vi "Link Bone Communication.vi"(6 "VISA resource name":refnum<visa-resource-name>="COM3", 8 "error in":errorcluster, 11 "Commands":string[](array[string])=["reset", "on A, I", "on B, J", "on C, K"]) -> (0 "error out":errorcluster)   [LabVIEW 2012]
uses:
  <vilib>/Instr/_visa.llb/VISA Configure Serial Port (Instr).vi
panel:
  out "read buffer":string
  out "Numeric":i32
  out "concatenated string":string
  out "bytes read":u32
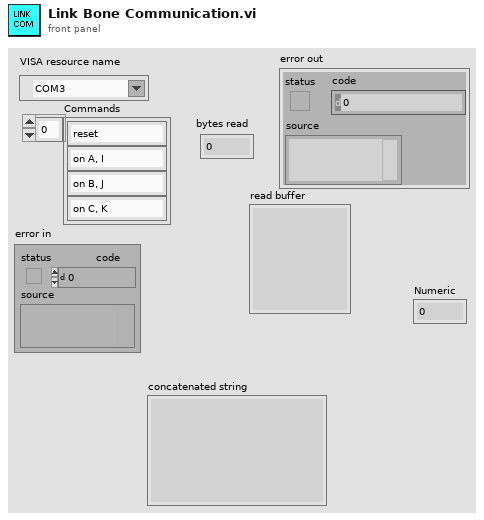
[diagram p1: front panel]
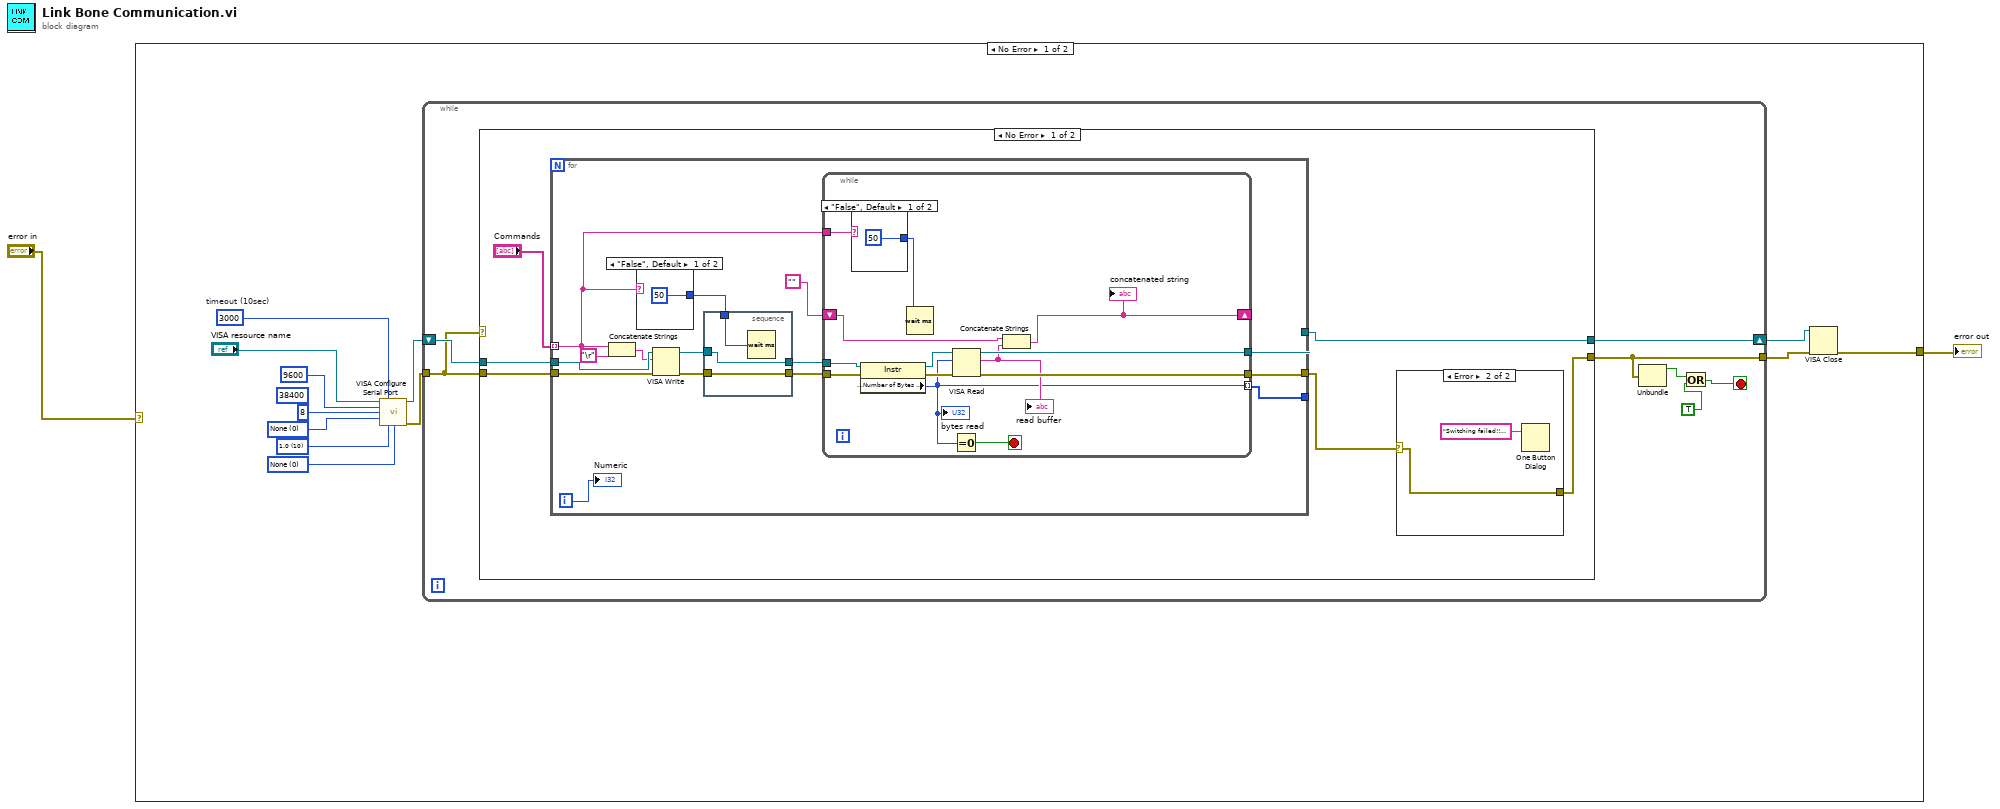
[diagram p0: block diagram]
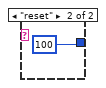
[diagram p3: hidden frame]
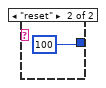
[diagram p4: hidden frame]
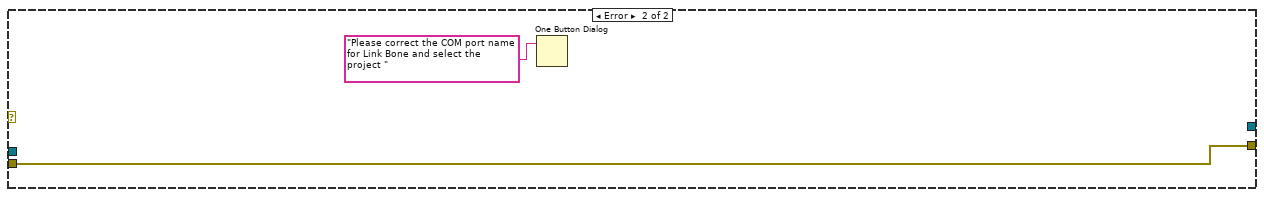
[diagram p5: hidden frame]
diagram:
  n1 = case shown="No Error" "error in" {
    selector: "error in" -> [_ w68]
    tunnel: [w3 w68] -> w1
    frame No Error {
      w6 = u16 0 items=["None"=0, "XON/XOFF"=1, "RTS/CTS"=2, "DTR/DSR"=4] ("flow control")
      w7 = u16 10 items=["1.0"=10, "1.5"=15, "2.0"=20] ("stop bits")
      w9 = u16 0 items=["None", "Odd", "Even", "Mark", "Space"] ("parity")
      (unwired) u32 38400 ("baud rate")
      w8 = u32 3000  # timeout (10sec)
      n2 = call-poly "VISA Configure Serial Port"("VISA resource name"="VISA resource name", "timeout (10sec)"=w8, "baud rate (9600)"=u32 9600 ("baud rate"), "data bits (8)"=u16 8 ("data bits"), "parity (0:none)"=w9, "stop bits (10: 1 bit)"=w7, "flow control (0:none)"=w6) -> ("VISA resource name out"=w12:refnum<visa-resource-name>, "error out"=w13:errorcluster)  [unwired: 2 in, 5 out]
      n3 = while {
        tunnel: w13 -> [w16]
        tunnel: [w15] -> w11
        shift-right: [w20] -> w10
        shift-left: w12 -> [w21]
        stop <- w18 stop-if-true
        n4 = case shown="No Error" w16 {
          tunnel: w16 -> [w27 w66]
          tunnel: w21 -> [w26 _]
          tunnel: [w25 _] -> w20
          tunnel: [w23 w66] -> w15
          frame No Error {
            n5 = for {
              tunnel: w27 -> [w45]
              tunnel: w26 -> [w44]
              tunnel: [w31] -> w22
              tunnel: [w43] -> w25
              tunnel: "Commands" -> [w33] mode=indexing
              tunnel: [w32] -> _
              i -> [w35]
              n6 = Concatenate Strings(w33, "\r") -> (w37:string)
              n7 = case shown="\"False\", Default" w33 {
                tunnel: [u32 50 ("delay before read (ms)") u32 100 ("delay before read (ms)")] -> w34
                frame "False", Default {
                }
                frame "reset" {
                }
              }
              n8 = VISA Write(VISA resource name=w44, write buffer=w37, error in (no error)=w45) -> (VISA resource name out=w40:refnum<visa-resource-name>, error out=w42:errorcluster)  [unwired: 1 out]
              n9 = stacked-sequence {
                tunnel: w42 -> [w65]
                tunnel: [w65] -> w41
                tunnel: w40 -> [w64]
                tunnel: [w64] -> w39
                tunnel: w34 -> [w63]
                frame #0 {
                  n10 = Wait (ms)(milliseconds to wait=w63) -> ()  [unwired: 1 out]
                }
              }
              n11 = while {
                tunnel: [w60] -> w31
                tunnel: [w59] -> w43
                tunnel: w41 -> [w58]
                tunnel: w39 -> [w57]
                shift-right: [w51] -> _
                shift-left: "" -> [w53]
                tunnel: w33 -> [w49]
                tunnel: [w48] -> w32 mode=indexing
                stop <- w54 stop-if-true
                n12 = case shown="\"False\", Default" w49 {
                  tunnel: [u32 50 ("delay before read (ms)") u32 100 ("delay before read (ms)")] -> w50
                  frame "False", Default {
                  }
                  frame "reset" {
                  }
                }
                n13 = property class="Instr"(reference=w57, error in=w58) -> (reference out=w56:refnum<visa-resource-name>, error out=w55:errorcluster, "Serial Settings:Number of Bytes at Serial Port"=w48:u32)
                "bytes read" <- w48
                n14 = Wait (ms)(milliseconds to wait=w50) -> ()  [unwired: 1 out]
                n15 = VISA Read(VISA resource name=w56, byte count=w48, error in (no error)=w55) -> (VISA resource name out=w59:refnum<visa-resource-name>, read buffer=w52:string, error out=w60:errorcluster)  [unwired: 1 out]
                "read buffer" <- w52
                n16 = Equal To 0?(x=w48) -> (x = 0?=w54:bool)
                n17 = Concatenate Strings(w53, w52) -> (w51:string)
                "concatenated string" <- w51
              }
              "Numeric" <- w35
            }
            n18 = case shown="Error" w22 {
              selector: w22 -> [w28 w29]
              tunnel: [w28 w29] -> w23
              frame No Error {
              }
              frame Error {
                n19 = One Button Dialog(message="Switching failed!! please check the link bone is switched ON or serial port is connected") -> ()  [unwired: 1 in, 1 out]
              }
            }
          }
          frame Error {
            n20 = One Button Dialog(message="Please correct the COM port name for Link Bone and select the project ") -> ()  [unwired: 1 in, 1 out]
          }
        }
        n21 = Unbundle(w15) -> ("status"=w19:bool)  [unwired: 2 out]
        n22 = Or(x=w19, y=TRUE) -> (x .or. y?=w18:bool)
      }
      n23 = VISA Close(VISA resource name=w10, error in (no error)=w11) -> (error out=w3:errorcluster)
    }
    frame Error {
    }
  }
  "error out" <- w1
